vi "ResponseStreaming RouteGuide Test.vi"(11 "Request Data":T3) -> (0 "error out":errorcluster, 3 "Response Data":T1[](array[typedef]))   [LabVIEW 2019, in "route_guide_client.lvlib"]
uses:
  route_guide_client.lvlib
  RPC Messages/routeguide_Rectangle.ctl
  RPC Messages/routeguide_Point.ctl
  RPC Messages/routeguide_Feature.ctl
panel:
  in  "error in":errorcluster
  in  "Server Address":string="localhost:50051"
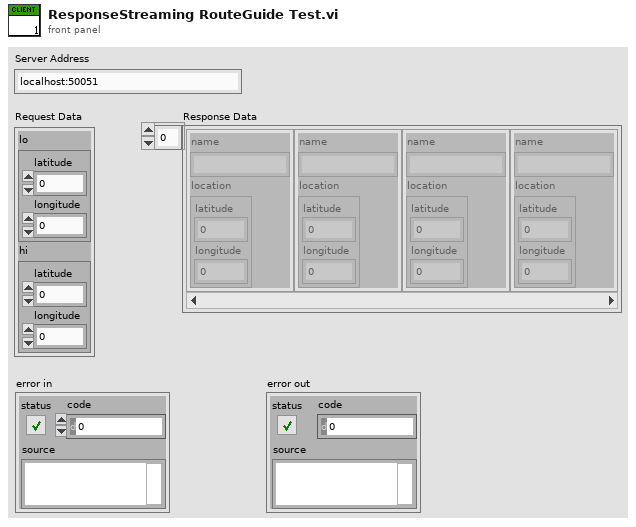
[diagram p1: front panel]
types:
  T1 = typedef "route_guide_client.lvlib/routeguide_Feature.ctl" = cluster{"name":string, "location":T2}
  T2 = typedef "route_guide_client.lvlib/routeguide_Point.ctl" = cluster{"latitude":i32, "longitude":i32}
  T3 = typedef "route_guide_client.lvlib/routeguide_Rectangle.ctl" = cluster{"lo":T2, "hi":T2}
  T4 = typedef "grpc-lvsupport-release.lvlib/grpcId.ctl" = u64
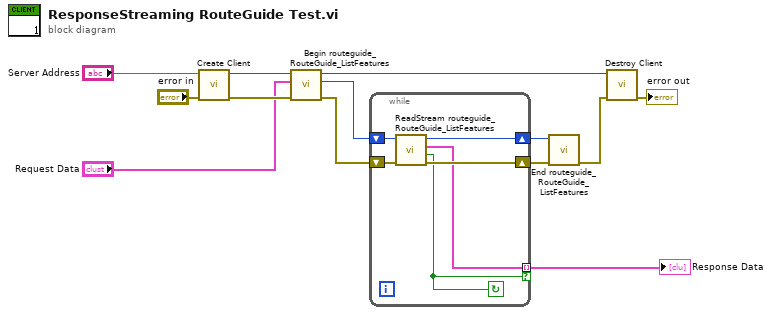
[diagram p0: block diagram]
diagram:
  n1 = call "Create Client.vi"("error in"="error in", "address"="Server Address") -> ("error out"=w11:errorcluster, "gRPC ID Out"=w12:T4)  [unwired: 8 in]
  n2 = call "Begin routeguide_RouteGuide_ListFeatures.vi"("error in"=w11, "Request Data"="Request Data", "gRPC ID"=w12) -> ("error out"=w9:errorcluster, "Call Id Out"=w8:T4, "gRPC ID out"=w5:T4)  [unwired: 6 in]
  n3 = while {
    shift-right: [w16] -> w6
    shift-left: w9 -> [w19]
    shift-right: [w17] -> w7
    shift-left: w8 -> [w18]
    tunnel: [w15] -> w3 mode=indexing if=w14
    stop <- w14 continue-if-true
    n4 = call "ReadStream routeguide_RouteGuide_ListFeatures.vi"("error in"=w19, "Call ID in"=w18) -> ("error out"=w16:errorcluster, "Success"=w14:bool, "Response Data"=w15:T1, "Call ID"=w17:T4)  [unwired: 6 in]
  }
  "Response Data" <- w3
  n5 = call "End routeguide_RouteGuide_ListFeatures.vi"("error in"=w6, "Call ID in"=w7) -> ("error out"=w4:errorcluster)  [unwired: 8 in, 1 out]
  n6 = call "Destroy Client.vi"("error in"=w4, "gRPC ID"=w5) -> ("error out"=→"error out":errorcluster)  [unwired: 9 in]
